vi "Global 1.vi"() -> ()   [LabVIEW 2017]
panel:
  out "Loop Time PLC 8":u8
  out "Loop Time PLC 7":u8
  out "Loop Time PLC 6":u8
  out "Loop Time PLC 5":u8
  out "Loop Time PLC 4":u8
  out "Loop Time PLC 3":u8
  out "Loop Time PLC 2":u8
  out "Loop Time PLC 1":u8
  out "PLC8 error":errorcluster
  out "PLC7 error":errorcluster
  out "PLC6 error":errorcluster
  out "PLC5 error":errorcluster
  out "PLC4 error":errorcluster
  out "PLC3 error":errorcluster
  out "PLC2 error":errorcluster
  out "PLC1 error":errorcluster
  out "PLC 8":bool
  in  "Filtered BARCODE selected":string[](array[string])
  out "PLC 7":bool
  out "PLC 6":bool
  out "PLC 5":bool
  out "RESET TRIGGER OP60":bool
  in  "FOR COMARISION":string
  out "send data to plc":bool
  in  "OP 60 BARCODE SEND TO PLC":string
  out "STATION 2 OK":bool
  out "EMERGENCY STOP":bool
  in  "LASER DATA FOR PLC":string
  in  "OP 60 BARCODE":string
  in  "BARCODE RECIPE":string
  out "RECHECK RESULT OK":bool
  out "PLC 4":bool
  out "PLC 3":bool
  out "PLC 2":bool
  out "PLC 1":bool
  out "RESET FOR PRINT":bool
  out "BOM ALARM LAST2 ST 5":bool
  out "BOM ALARM LAST ST 5":bool
  out "BOM ALARM LAST2 ST 4":bool
  out "BOM ALARM LAST ST 4":bool
  out "BOM ALARM LAST2 ST 3":bool
  out "BOM ALARM LAST ST 3":bool
  out "BOM ALARM LAST2 ST 2":bool
  out "BOM ALARM LAST ST 2":bool
  out "PLC COMM":bool
  out "BOM ALARM LAST2 ST 1":bool
  out "BOM ALARM LAST ST 1":bool
  out "CYCLE START 6":bool
  out "CYCLE START 5":bool
  out "CYCLE START 4":bool
  out "CYCLE START 3":bool
  out "CYCLE START 2":bool
  out "CYCLE START 1":bool
  in  "result6":bool
  in  "result5":bool
  in  "result4":bool
  in  "result3":bool
  in  "result2":bool
  in  "result1":bool
  in  "scanner 6":string
  in  "scanner 5":string
  in  "scanner 4":string
  in  "scanner 3":string
  in  "scanner 2":string
  in  "scanner 1":string
  in  "RECIPE NAME":string
  out "MODEL SELECTION":bool
  out "REMOVE VI":bool
  out "REMOVE VI SUBPANEL SETTING":bool
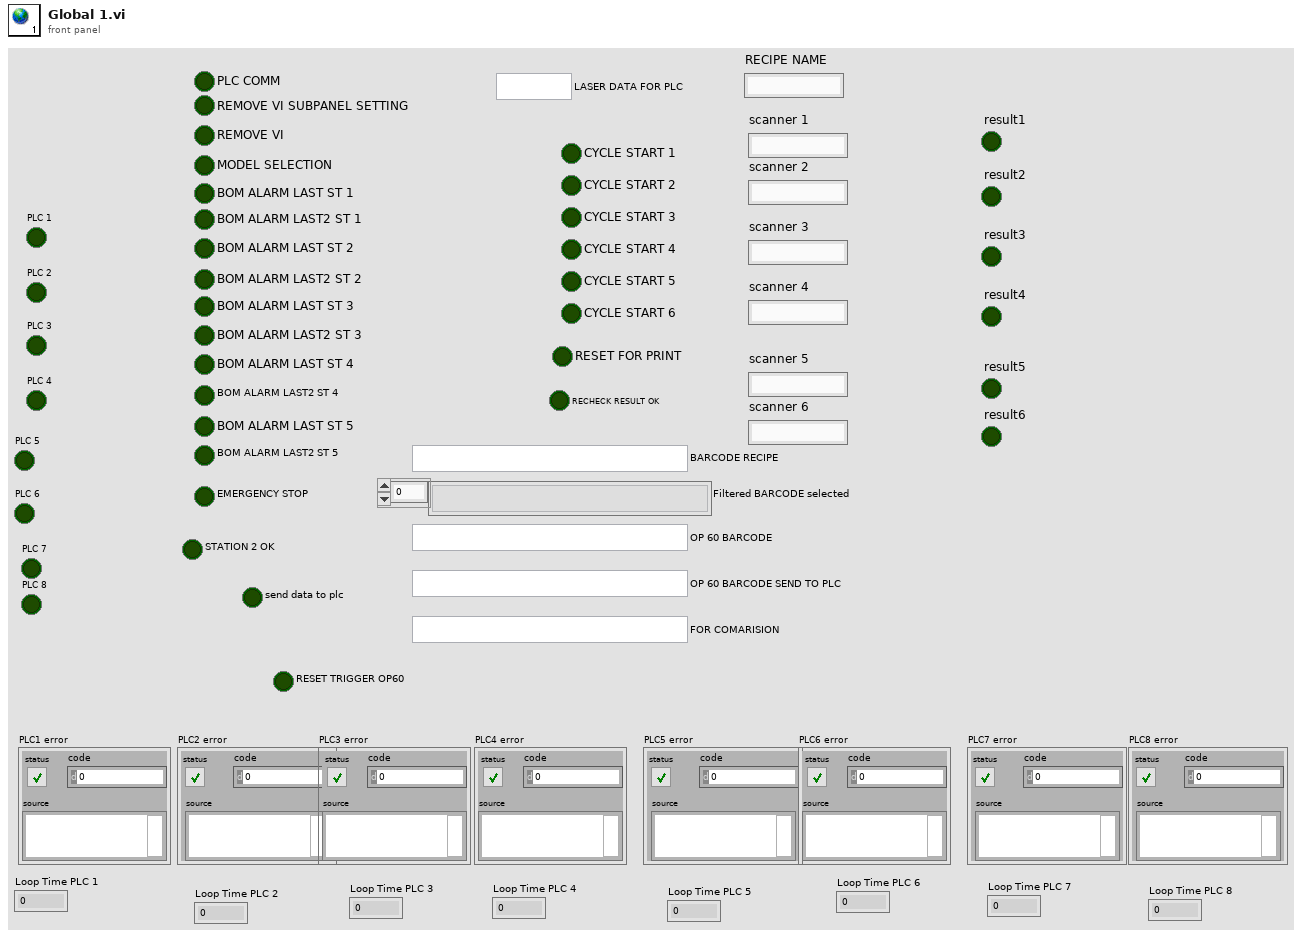
[diagram p1: front panel]
diagram:
